vi "Check Versions.vi"(6 "Error Message in":string, 8 "Error In":errorcluster, 10 "Local Version Array":i32[](array[numeric]), 11 "Server Files Cluster":T1) -> (0 "Error Out":errorcluster, 3 "Update Files":bool, 4 "Error Message out":string)   [LabVIEW 2019]
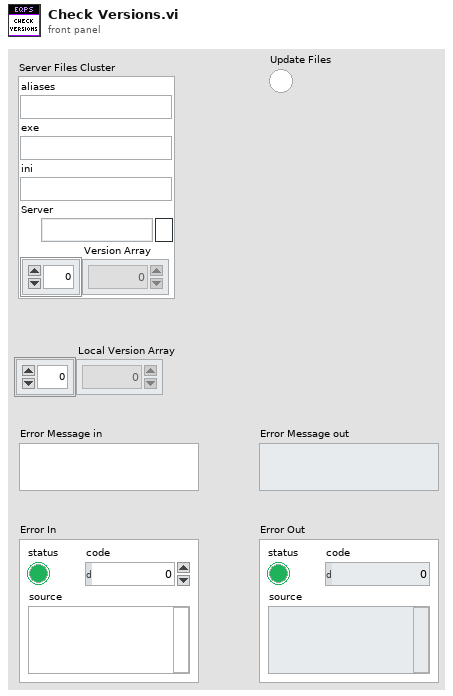
[diagram p1: front panel]
types:
  T1 = cluster{"aliases":string, "exe":string, "ini":string, "Server":path, "Version Array":i32[]}
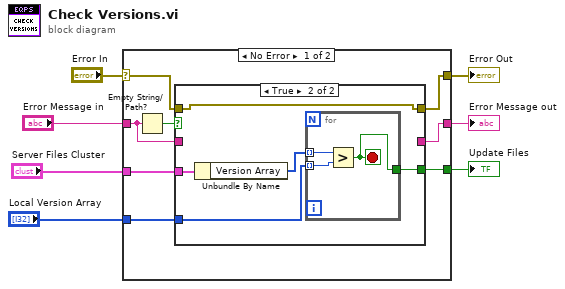
[diagram p0: block diagram]
diagram:
  n1 = case shown="No Error" "Error In" {
    selector: "Error In" -> [w11 w27]
    tunnel: [w12 w27] -> w6
    tunnel: [w14 w26] -> w5
    tunnel: "Error Message in" -> [w13 w26]
    tunnel: "Server Files Cluster" -> [w10 _]
    tunnel: "Local Version Array" -> [w9 _]
    tunnel: [w8 _] -> w1
    frame No Error {
      n2 = Empty String/Path?(string/path=w13) -> (empty?=w15:bool)
      n3 = case shown="True" w15 {
        tunnel: [w17 _] -> w14
        tunnel: w13 -> [w17 _]
        tunnel: [w16 w21] -> w12
        tunnel: w11 -> [w16 w21]
        tunnel: w10 -> [_ w22]
        tunnel: w9 -> [_ w19]
        tunnel: [_ w18] -> w8
        frame False {
        }
        frame True {
          n4 = Unbundle By Name(w22) -> ("Version Array"=w20:i32[])
          n5 = for {
            tunnel: w20 -> [w25] mode=indexing
            tunnel: w19 -> [w24] mode=indexing
            tunnel: [w23] -> w18
            stop <- w23 stop-if-true
            n6 = Greater?(x=w25, y=w24) -> (0:w23:bool)
          }
        }
      }
    }
    frame Error {
    }
  }
  "Error Out" <- w6
  "Error Message out" <- w5
  "Update Files" <- w1
